vi "传感器数据.vi"() -> (3 "传感器读数":T1 {"吸收电流" format="%#.3f"; "输出扭矩(大)" format="%#.3f"; "输出扭矩(小)" format="%#.3f"; "输入扭矩" format="%#.3f"; "输入编码位移" format="%#.3f"; "工装移载位移" format="%#.3f"; "输入移载位移" format="%#.3f"; "输入旋转位移" format="%#.3f"})   [LabVIEW 2020]
uses:
  Libraries/S7/S7.lvlib
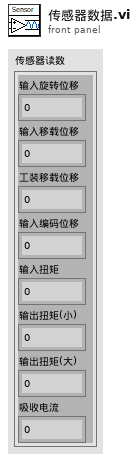
[diagram p1: front panel]
types:
  T1 = cluster{"输入旋转位移":sgl, "输入移载位移":sgl, "工装移载位移":sgl, "输入编码位移":sgl, "输入扭矩":sgl, "输出扭矩(小)":sgl, "输出扭矩(大)":sgl, "吸收电流":sgl}
  T2 = cluster{"输入轴扭矩":dbl, "输出轴扭矩小量程":dbl, "输出轴扭矩大量程":dbl}
  T3 = typedef "S7.lvlib/Read_Data (Reply Payload)--cluster.ctl" = cluster{"读取成功":bool, "数据":u32[], "Read_Data_error":errorcluster}
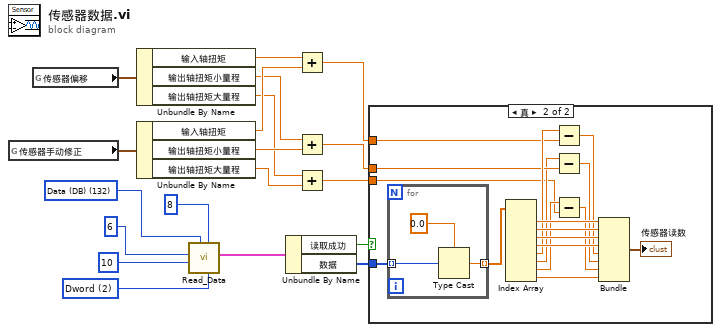
[diagram p0: block diagram]
diagram:
  w16 = u16 2 items=["byte", "word", "Dword"] ("数据类型")
  w17 = u8 132 items=["I/O (P)"=128, "Input (I)"=129, "Output (Q)"=130, "Bit Memory (M)"=131, "Data (DB)"=132, "Instance Data (DI)"=133, "Local Data (L)"=134, "Predecessor Local Data (VL)"=135] ("寄存器类型")
  n1 = global read "传感器偏移.vi" "传感器手动修正"() -> (w10:T2)
  n2 = global read "传感器偏移.vi" "传感器偏移"() -> (w11:T2)
  n3 = Unbundle By Name(w11) -> ("输入轴扭矩"=w9:dbl, "输出轴扭矩小量程"=w7:dbl, "输出轴扭矩大量程"=w5:dbl)
  n4 = Unbundle By Name(w10) -> ("输入轴扭矩"=w8:dbl, "输出轴扭矩小量程"=w6:dbl, "输出轴扭矩大量程"=w4:dbl)
  n5 = call "Read_Data.vi"("数据类型"=w16, "读取长度"=u16 8, "寄存器类型"=w17, "起始地址"=u32 10, "DB #"=u16 6) -> ("Reply Payload"=w14:T3)  [unwired: 4 in, 2 out]
  n6 = Unbundle By Name(w14) -> ("读取成功"=w12:bool, "数据"=w13:u32[])
  n7 = Add(x=w9, y=w8) -> (x+y=w3:dbl)
  n8 = Add(x=w7, y=w6) -> (x+y=w2:dbl)
  n9 = Add(x=w5, y=w4) -> (x+y=w1:dbl)
  n10 = case shown="真" w12 {
    tunnel: w13 -> [_ w36]
    tunnel: w3 -> [_ w26]
    tunnel: w2 -> [_ w25]
    tunnel: w1 -> [_ w21]
    frame False {
    }
    frame True {
      n11 = for {
        tunnel: w36 -> [w38] mode=indexing
        tunnel: [w37] -> w35 mode=indexing
        n12 = Type Cast(type=sgl 0.0, x=w38) -> (*(type *) &x=w37:sgl)
      }
      n13 = Index Array(array=w35) -> (element #1=w34:sgl, element #2=w33:sgl, element #3=w32:sgl, element #4=w31:sgl, element #5=w30:sgl, element #6=w24:sgl, element #7=w22:sgl, element #8=w29:sgl)  [unwired: 8 in]
      n14 = Subtract(x=w30, y=w26) -> (x-y=w27:dbl)
      n15 = Subtract(x=w24, y=w25) -> (x-y=w23:dbl)
      n16 = Subtract(x=w22, y=w21) -> (x-y=w20:dbl)
      n17 = Bundle(w34, w33, w32, w31, w27, w23, w20, w29) -> (→"传感器读数":cluster{sgl, sgl, sgl, sgl, dbl, dbl, dbl, sgl})  [unwired: 1 in]
    }
  }
